vi "Get Relative Path for Dependency.vi"(0 "Old measurement path":path, 5 "Old dependency path":path, 7 "New dependency path":path, 11 "error in (no error)":errorcluster) -> (4 "Dependency directory path":path, 15 "error out":errorcluster)   [LabVIEW 2021, in "Multiple Converter.lvlib"]
uses:
  Multiple Converter.lvlib
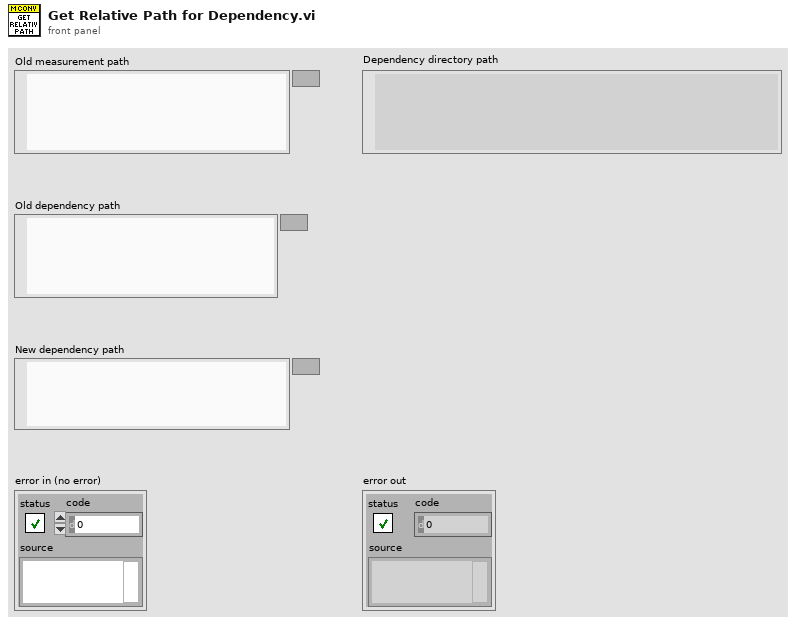
[diagram p1: front panel]
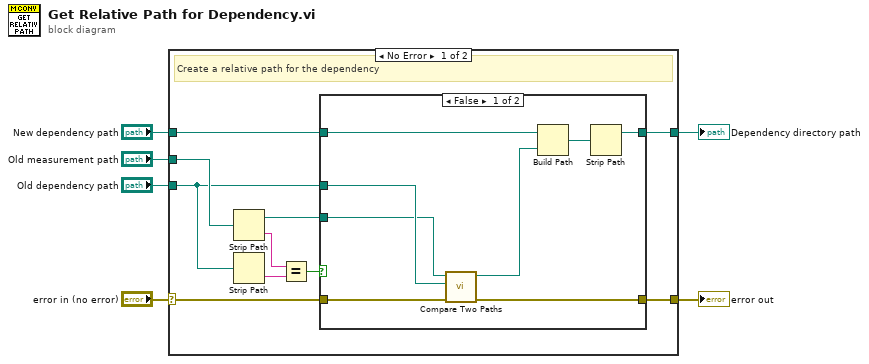
[diagram p0: block diagram]
diagram:
  n1 = case shown="No Error" "error in (no error)" {
    selector: "error in (no error)" -> [w9 w27]
    tunnel: "New dependency path" -> [w16 _]
    tunnel: [w15 _] -> w5
    tunnel: "Old measurement path" -> [w14 _]
    tunnel: "Old dependency path" -> [w13 _]
    tunnel: [w8 w27] -> w1
    frame No Error {
      # "Create a relative path for the dependency"
      n2 = Strip Path(path=w14) -> (stripped path=w7:path, name=w12:string)
      n3 = Strip Path(path=w13) -> (name=w11:string)  [unwired: 1 out]
      n4 = Equal?(x=w12, y=w11) -> (x = y?=w10:bool)
      n5 = case shown="False" w10 {
        tunnel: w16 -> [w24 w26]
        tunnel: [w22 w26] -> w15
        tunnel: w13 -> [w21 _]
        tunnel: w9 -> [w19 w25]
        tunnel: [w18 w25] -> w8
        tunnel: w7 -> [w17 _]
        frame False {
          n6 = call <vilib>:"Compare Two Paths.vi"("error in (no error)"=w19, "Path 2"=w21, "Path 1"=w17) -> ("error out"=w18:errorcluster, "Relative Path from 1 to 2"=w20:path)  [unwired: 5 in, 2 out]
          n7 = Build Path(base path=w24, name or relative path=w20) -> (appended path=w23:path)
          n8 = Strip Path(path=w23) -> (stripped path=w22:path)  [unwired: 1 out]
        }
        frame True {
        }
      }
    }
    frame Error {
    }
  }
  "Dependency directory path" <- w5
  "error out" <- w1
